vi "TCF to Dictionaries.vi"(8 "error in (no error)":errorcluster, 11 "QPA TCF Parser in":refnum<class "QPA TCF Parser.lvclass">) -> (0 "error out":errorcluster, 2 "Dictionaries Out":refnum<class "String Database.lvclass">[](array[class]), 3 "QPA TCF Parser out":refnum<class "QPA TCF Parser.lvclass">)   [LabVIEW 2016, in "QPA TCF Parser.lvlib" / "QPA TCF Parser.lvclass"]
uses:
  QPA TCF Parser.lvclass
  Plugins/String Database.lvlibp/String Database.lvclass
  QPA TCF Parser.lvclass/QPA TCF Parser.ctl
  Accessors/Read TCF Data.vi
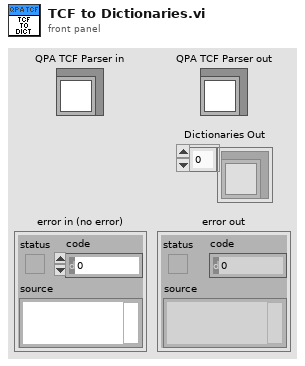
[diagram p1: front panel]
types:
  T1 = typedef "QPA TCF Parser.lvlib/QPA TCF Parser.lvclass/Worksheet Data.ctl" = cluster{"Worksheet Name":string, "Worksheet Data":string[][]}
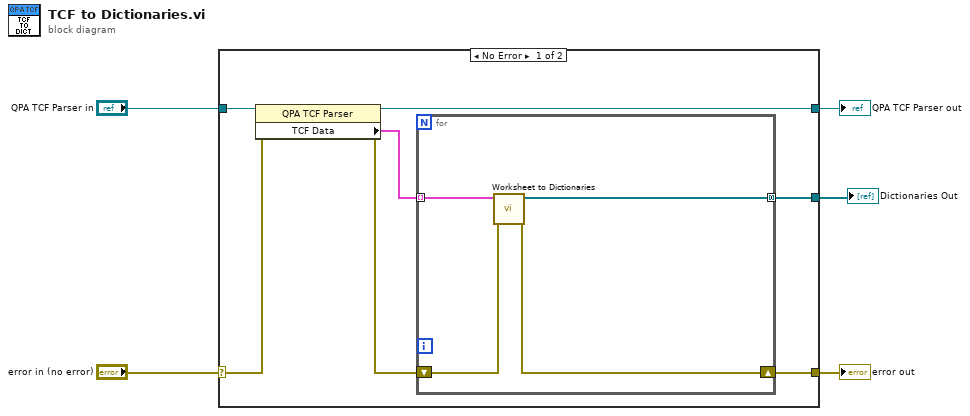
[diagram p0: block diagram]
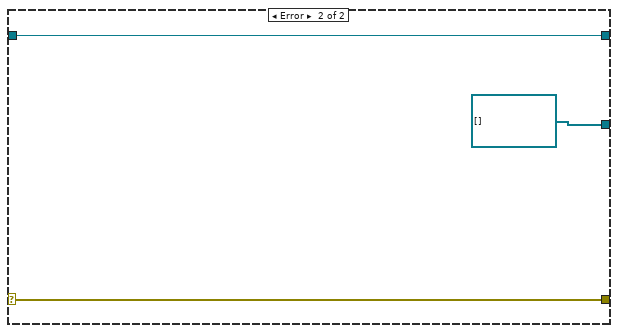
[diagram p2: hidden frame]
diagram:
  n1 = case shown="No Error" "error in (no error)" {
    selector: "error in (no error)" -> [w12 w19]
    tunnel: [w7 w19] -> w4
    tunnel: [w10 w18] -> w2
    tunnel: "QPA TCF Parser in" -> [w11 w18]
    tunnel: [w6 refnum<class "String Database.lvclass">[] [] ("Dictionaries Out")] -> w1
    frame No Error {
      n2 = property class="QPA TCF Parser"(reference=w11, error in=w12) -> (reference out=w10:refnum<class "QPA TCF Parser.lvclass">, error out=w8:errorcluster, "TCF Data"=w9:T1[])
      n3 = for {
        tunnel: w9 -> [w16] mode=indexing
        shift-right: [w14] -> w7
        shift-left: w8 -> [w15]
        tunnel: [w13] -> w6 mode=concatenating
        n4 = call "Worksheet to Dictionaries.vi"("error in (no error)"=w15, "Worksheet Data"=w16) -> ("error out"=w14:errorcluster, "Dictionaries Out"=w13:refnum<class "String Database.lvclass">[])  [unwired: 8 in]
      }
    }
    frame Error {
    }
  }
  "error out" <- w4
  "QPA TCF Parser out" <- w2
  "Dictionaries Out" <- w1
